vi "LoadChosenDevice.vi"(4 "error in (no error)":errorcluster, 7 "Chosen Device":T1) -> (0 "error out":errorcluster, 3 "Loaded Device":refnum<class "Device.lvclass">)   [LabVIEW 2013]
uses:
  Device/Device.lvclass
  Master Device/Master Device.lvclass
  <vilib>/Utility/error.llb/DialogType.ctl
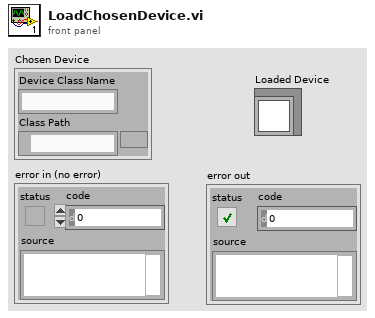
[diagram p1: front panel]
types:
  T1 = cluster{"Device Class Name":string, "Class Path":path}
  T2 = typedef "DialogType.ctl" = u16
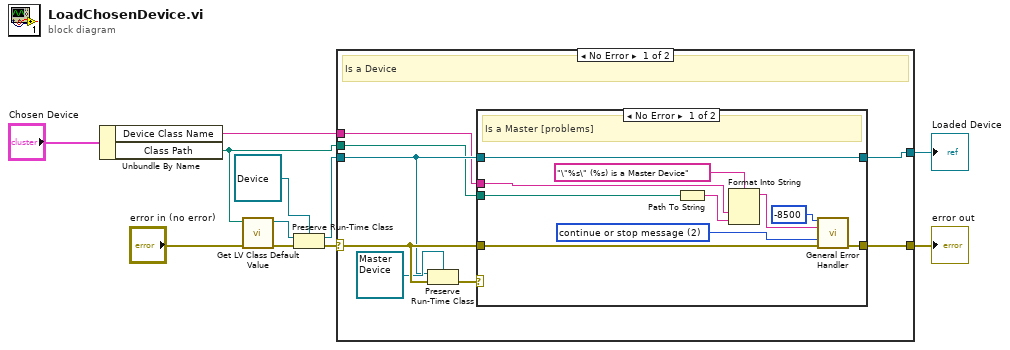
[diagram p0: block diagram]
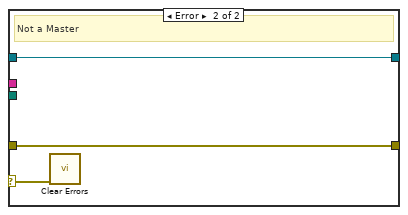
[diagram p2: hidden frame]
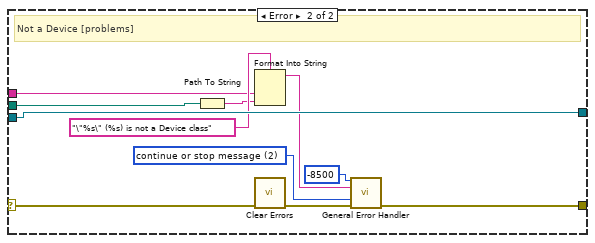
[diagram p3: hidden frame]
diagram:
  n1 = Unbundle By Name("Chosen Device") -> ("Device Class Name"=w2:string, "Class Path"=w1:path)
  n2 = call <vilib>:"Get LV Class Default Value.vi"("error in (no error)"="error in (no error)", "class path"=w1) -> ("error out"=w8:errorcluster, "object"=w9:refnum<class>)  [unwired: 8 in]
  n3 = Preserve Run-Time Class(object in=w9, error in=w8, 2:refnum<class "Device.lvclass"> refnum ("Device.lvclass")) -> (object out=w11:refnum<class "Device.lvclass">, error out=w10:errorcluster)
  n4 = case shown="No Error" w10 {
    selector: w10 -> [w17 w38]
    tunnel: w11 -> [w15 w43]
    tunnel: [w18 w36] -> w5
    tunnel: [w14 w43] -> w6
    tunnel: w2 -> [w13 w35]
    tunnel: w1 -> [w12 w34]
    frame No Error {
      # "Is a Device"
      n5 = Preserve Run-Time Class(object in=w15, error in=w17, 2:refnum<class "Master Device.lvclass"> refnum ("Master Device.lvclass")) -> (error out=w19:errorcluster)  [unwired: 1 out]
      n6 = case shown="No Error" w19 {
        selector: w19 -> [_ w32]
        tunnel: [w28 w31] -> w18
        tunnel: w17 -> [w29 w31]
        tunnel: w15 -> [w27 w30]
        tunnel: [w27 w30] -> w14
        tunnel: w13 -> [w23 _]
        tunnel: w12 -> [w21 _]
        frame No Error {
          w25 = T2 2 items=["no dialog", "OK message", "continue or stop message", "OK message + warnings", "continue/stop + warnings"] ("type of dialog (OK msg:1)")
          # "Is a Master [problems]"
          n7 = Path To String(path=w21) -> (string=w20:string)
          n8 = Format Into String(format string="\"%s\" (%s) is a Master Device", w23, w20) -> (resulting string=w22:string)  [unwired: 2 in, 1 out]
          n9 = call <vilib>:"General Error Handler.vi"("[error code] (0)"=-8500, "[error source] (\" \")"=w22, "type of dialog (OK msg:1)"=w25, "error in (no error)"=w29) -> ("error out"=w28:errorcluster)  [unwired: 7 in, 4 out]
        }
        frame Error {
          # "Not a Master"
          n10 = call <vilib>:"Clear Errors.vi"("error in (no error)"=w32) -> ()  [unwired: 6 in, 1 out]
        }
      }
    }
    frame Error {
      w41 = T2 2 items=["no dialog", "OK message", "continue or stop message", "OK message + warnings", "continue/stop + warnings"] ("type of dialog (OK msg:1)")
      # "Not a Device [problems]"
      n11 = Path To String(path=w34) -> (string=w33:string)
      n12 = Format Into String(format string="\"%s\" (%s) is not a Device class", w35, w33) -> (resulting string=w39:string)  [unwired: 2 in, 1 out]
      n13 = call <vilib>:"Clear Errors.vi"("error in (no error)"=w38) -> ("error out"=w37:errorcluster)  [unwired: 6 in]
      n14 = call <vilib>:"General Error Handler.vi"("[error code] (0)"=-8500, "[error source] (\" \")"=w39, "type of dialog (OK msg:1)"=w41, "error in (no error)"=w37) -> ("error out"=w36:errorcluster)  [unwired: 7 in, 4 out]
    }
  }
  "Loaded Device" <- w6
  "error out" <- w5
